vi "createDeviceData.vi"(8 "error in (no error)":errorcluster, 11 "DoDeviceData in":refnum<class "DoDeviceData.lvclass">) -> (0 "error out":errorcluster, 3 "DoDeviceData out":refnum<class "DoDeviceData.lvclass">)   [LabVIEW 2011, in "DataMappers.lvlib" / "DoDeviceData.lvclass"]
uses:
  DoDeviceData.lvclass
  Hal/Channels/Digital/DigitalOutput.lvclass
  DoDeviceData.lvclass/DoDeviceData.ctl
  DeviceData.lvclass
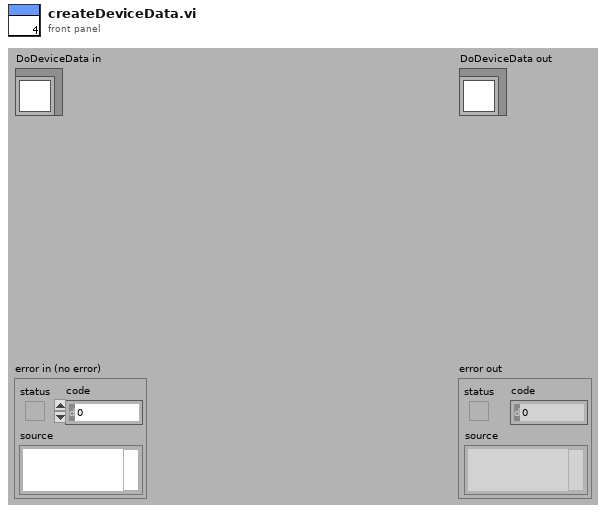
[diagram p1: front panel]
types:
  T1 = cluster{"Master Clock source":string, "Master Clock rate":dbl, "Start trigger line":string, "Scan rate":dbl, "Stop trigger line":string, "Sample Number":dbl}
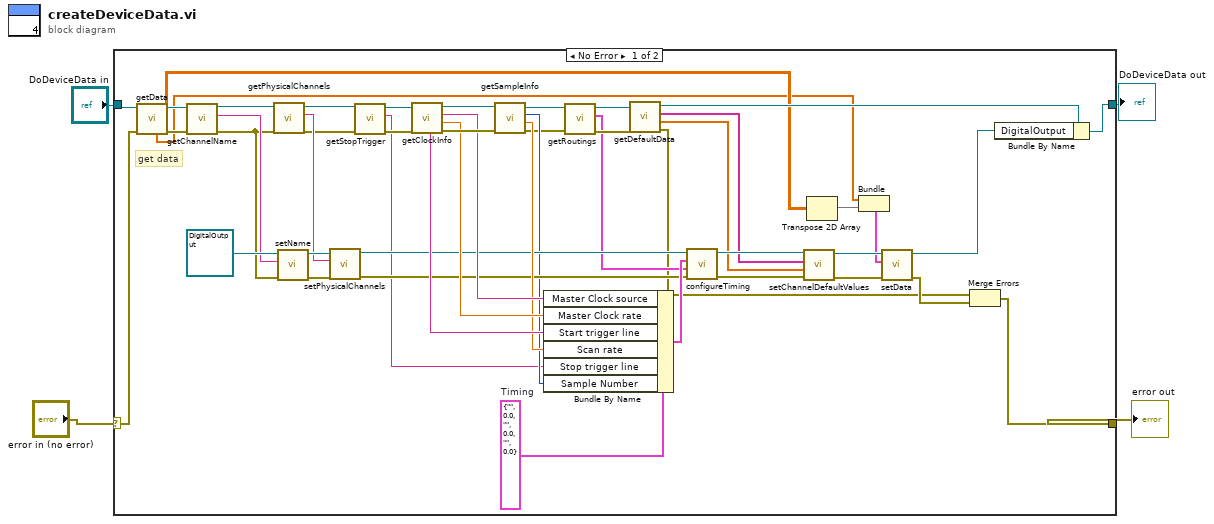
[diagram p0: block diagram]
diagram:
  n1 = case shown="No Error" "error in (no error)" {
    selector: "error in (no error)" -> [w8 w53]
    tunnel: [w44 w54] -> w1
    tunnel: "DoDeviceData in" -> [w9 w54]
    tunnel: [w45 w53] -> w2
    frame No Error {
      w34 = T1 {"Master Clock source"="", "Master Clock rate"=0.0, "Start trigger line"="", "Scan rate"=0.0, "Stop trigger line"="", "Sample Number"=0.0}  # Timing
      # "get data"
      n2 = call "getData.vi"("error in (no error)"=w8, "DeviceData in"=w9) -> ("error out"=w7:errorcluster, "dataArray"=w6:dbl[][], "DeviceData out"=w10:refnum<class "DoDeviceData.lvclass">, "times"=w5:dbl[])  [unwired: 4 in, 2 out]
      n3 = call "getChannelName.vi"("error in (no error)"=w7, "DeviceData in"=w10) -> ("error out"=w41:errorcluster, "channelName"=w42:string, "DeviceData out"=w52:refnum<class "DoDeviceData.lvclass">)  [unwired: 7 in]
      n4 = call "getPhysicalChannels.vi"("error in (no error)"=w41, "DeviceData in"=w52) -> ("error out"=w16:errorcluster, "physicalChannels"=w38:string, "DeviceData out"=w15:refnum<class "DoDeviceData.lvclass">)  [unwired: 7 in]
      n5 = call-dynamic "setName.vi"("error in (no error)"=w41, "name"=w42, "DigitalOutput.lvclass in"=refnum<class "DigitalOutput.lvclass"> refnum ("Hardware:Channels.lvlib:DigitalOutput.lvclass")) -> ("error out"=w39:errorcluster, "DigitalOutput.lvclass out"=w40:refnum<class "DigitalOutput.lvclass">)  [unwired: 7 in]
      n6 = call-dynamic "setPhysicalChannels.vi"("error in (no error)"=w39, "Physical Channels"=w38, "DigitalOutput.lvclass in"=w40) -> ("error out"=w35:errorcluster, "DigitalOutput.lvclass out"=w36:refnum<class "DigitalOutput.lvclass">)  [unwired: 7 in]
      n7 = call "getStopTrigger.vi"("error in (no error)"=w16, "DoDeviceData in"=w15) -> ("error out"=w17:errorcluster, "stop_Trigger"=w14:string, "DoDeviceData out"=w18:refnum<class "DoDeviceData.lvclass">)  [unwired: 7 in]
      n8 = call "getClockInfo.vi"("error in (no error)"=w17, "DeviceData in"=w18) -> ("error out"=w50:errorcluster, "masterClockRate"=w48:dbl, "clock"=w49:string, "DeviceData out"=w51:refnum<class "DoDeviceData.lvclass">, "start_trigger"=w47:string)  [unwired: 5 in]
      n9 = call-dynamic "getSampleInfo.vi"("error in (no error)"=w50, "DeviceData in"=w51) -> ("error out"=w20:errorcluster, "sampleRate"=w46:dbl, "sampleNumber"=w33:i32, "DeviceData out"=w23:refnum<class "DoDeviceData.lvclass">)  [unwired: 6 in]
      n10 = Bundle By Name(cluster=w34, "Master Clock source"=w49, "Master Clock rate"=w48, "Start trigger line"=w47, "Scan rate"=w46, "Stop trigger line"=w14, "Sample Number"=w33) -> (w37:T1)
      n11 = call "getRoutings.vi"("error in (no error)"=w20, "DoDeviceData in"=w23) -> ("error out"=w21:errorcluster, "Routings"=w19:cluster{"Master Clock Route":string[]}, "DoDeviceData out"=w22:refnum<class "DoDeviceData.lvclass">)  [unwired: 7 in]
      n12 = call "getDefaultData.vi"("error in (no error)"=w21, "DeviceData in"=w22) -> ("error out"=w11:errorcluster, "calibratedValues"=w27:dbl[], "channelAddresses"=w28:string[], "DeviceData out"=w12:refnum<class "DoDeviceData.lvclass">)  [unwired: 6 in]
      n13 = call-dynamic "configureTiming.vi"("error in (no error)"=w35, "Routings"=w19, "Timing"=w37, "DigitalOutput in"=w36) -> ("error out"=w30:errorcluster, "DigitalOutput out"=w32:refnum<class "DigitalOutput.lvclass">)  [unwired: 6 in]
      n14 = call-dynamic "setChannelDefaultValues.vi"("error in (no error)"=w30, "calibratedValues"=w27, "channel_addresses"=w28, "DigitalOutput in"=w32) -> ("error out"=w29:errorcluster, "DigitalOutput out"=w31:refnum<class "DigitalOutput.lvclass">)  [unwired: 6 in]
      n15 = Transpose 2D Array(2D array=w6) -> (transposed array=w13:dbl[][])
      n16 = Bundle("times"=w5, w13) -> (w26:cluster{"times":dbl[], dbl[][]})  [unwired: 1 in]
      n17 = call-dynamic "setData.vi"("error in (no error)"=w29, "Data"=w26, "DigitalOutput.lvclass in"=w31) -> ("error out"=w24:errorcluster, "DigitalOutput.lvclass out"=w25:refnum<class "DigitalOutput.lvclass">)  [unwired: 7 in]
      n18 = Merge Errors(w11, w24) -> (w45:errorcluster)
      n19 = Bundle By Name(cluster=w12, "DigitalOutput"=w25) -> (w44:refnum<class "DoDeviceData.lvclass">)
    }
    frame Error {
    }
  }
  "error out" <- w2
  "DoDeviceData out" <- w1
